vi "TagSyncFPGA.vi"() -> ()   [LabVIEW 2017]
uses:
  <vilib>/rvi/Emulation/niFpgaSctlEmulationGetInTimedLoop.vi
  <vilib>/rvi/Emulation/niFpgaProcessEmulError.vi
  <vilib>/rvi/Emulation/niFpgaGetClockAttributes.vi
  <vilib>/rvi/Emulation/niFpgaEmulationReportErrorSimple.vi
  <vilib>/rvi/Emulation/niFpgaCriticalErrorInLSC.vi
  <vilib>/rvi/eio/common/nirviEmuTemplateMethod_errors.vi
  <vilib>/eio/EIONode/EIONode.xnode
panel:
  in  "Sync Tagging":T1(tab)
  out "Minimum tagging period (pws)":u32=87
  out "Total tag data length (pws)":u32=86
  in  "TaggingPeriod (pws)":u32=100
  out "TagMarkerDuration (pws)":u16=10
  in  "PulseWidth (ms)":u32=10
  out "Tag data does NOT fit in period!!!":bool
  in  "Halt tagging":bool
  out "Tag monitor":i16(graph)
  in  "Enable monitoring":bool
  out "Current tag number":i32=665
  out "Tag data":bool[](array[boolean])=[TRUE, TRUE, TRUE, TRUE, TRUE, TRUE, TRUE, TRUE, TRUE, TRUE, FALSE, TRUE, FALSE, FALSE, FALSE, FALSE, FALSE, TRUE, FALSE, TRUE, FALSE, FALSE, FALSE, FALSE, FALSE, TRUE, FALSE, FALSE, FALSE, TRUE, FALSE, FALSE, FALSE, FALSE, FALSE, FALSE, FALSE, FALSE, FALSE, FALSE, FALSE, FALSE, FALSE, FALSE, FALSE, FALSE, FALSE, FALSE, FALSE, FALSE, FALSE, FALSE, FALSE, FALSE, FALSE, FALSE, FALSE, FALSE, FALSE, FALSE, FALSE, FALSE, FALSE, FALSE, FALSE, FALSE, FALSE, FALSE, FALSE, FALSE, FALSE, FALSE, FALSE, FALSE, FALSE, FALSE, TRUE, TRUE, TRUE, TRUE, TRUE, TRUE, TRUE, TRUE, TRUE, TRUE, FALSE, FALSE, FALSE, FALSE, FALSE, FALSE, FALSE, FALSE, FALSE, FALSE, FALSE, FALSE, FALSE, FALSE, FALSE, FALSE, FALSE, FALSE, FALSE, FALSE, FALSE, FALSE, FALSE, FALSE, FALSE, FALSE, FALSE, FALSE, FALSE, FALSE, FALSE, FALSE, FALSE, FALSE, FALSE, FALSE, FALSE, FALSE, FALSE, FALSE, FALSE, FALSE, FALSE, FALSE, FALSE, FALSE, FALSE, FALSE, FALSE, FALSE, FALSE, FALSE, FALSE, FALSE, FALSE, FALSE, FALSE, FALSE, FALSE, FALSE, FALSE, FALSE, FALSE, FALSE, FALSE, FALSE]
  out "SyncTagOutput":bool
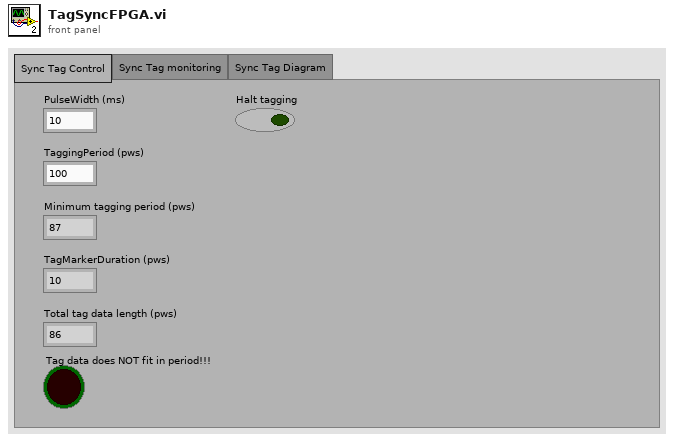
[diagram p1: front panel]
types:
  T1 = enum32{"Sync Tag Control", "Sync Tag monitoring", "Sync Tag Diagram"}
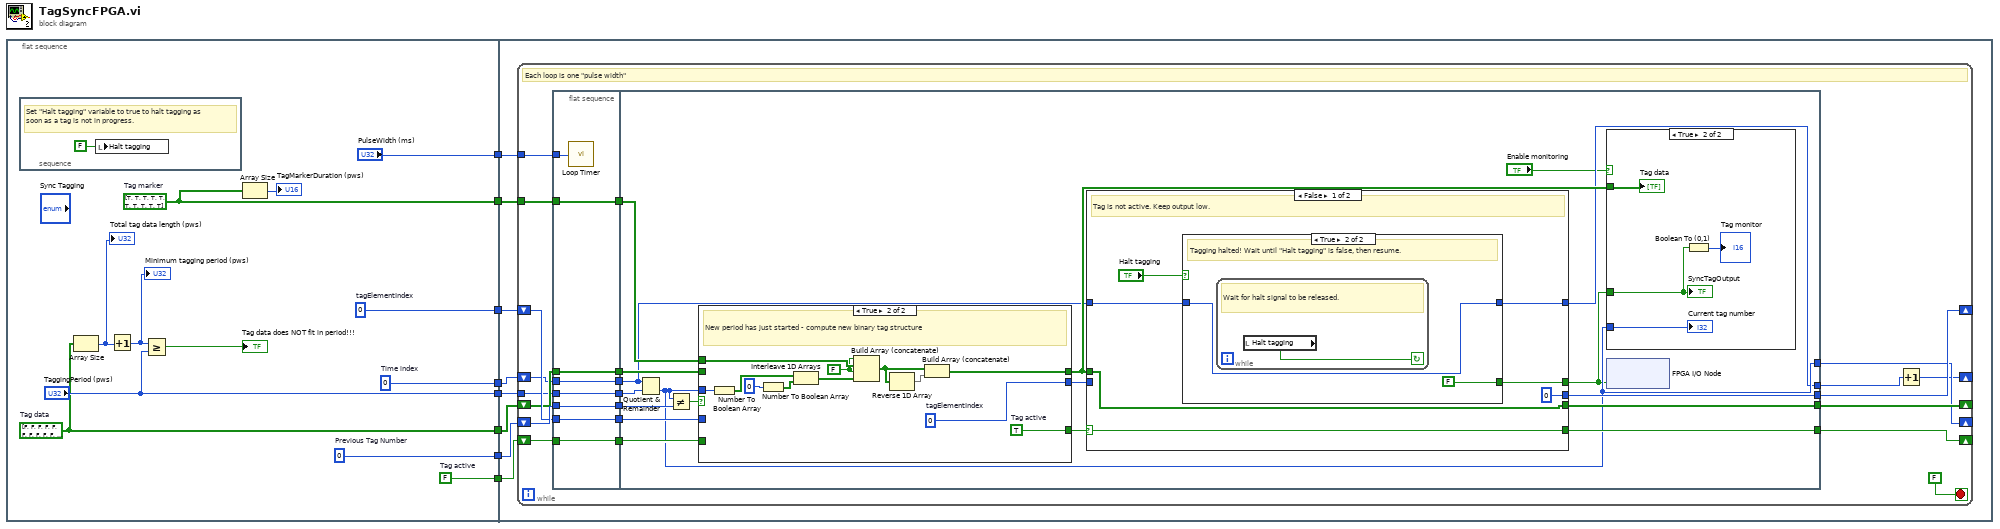
[diagram p0: block diagram]
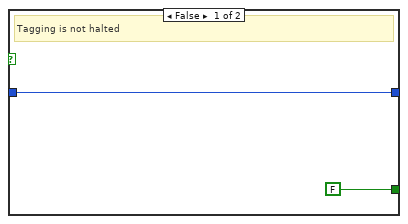
[diagram p3: hidden frame]
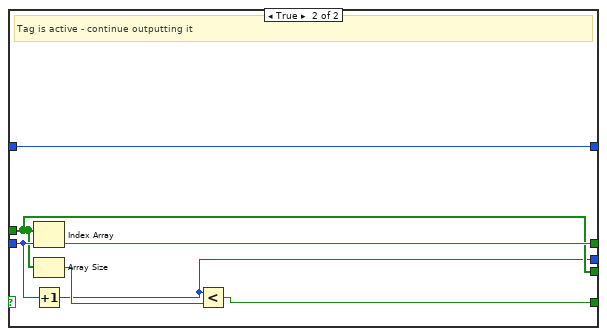
[diagram p4: hidden frame]
diagram:
  n1 = flat-sequence {
    tunnel: ["TaggingPeriod (pws)"] -> w8
    tunnel: [w19] -> w7
    tunnel: [w18] -> w6
    tunnel: [w17] -> w5
    tunnel: [w16] -> w4
    tunnel: [w15] -> w3
    tunnel: ["PulseWidth (ms)"] -> w2
    tunnel: [w13] -> w1
    tunnel: w8 -> [w25]
    tunnel: w7 -> [w24]
    tunnel: w6 -> [w28]
    tunnel: w5 -> [w26]
    tunnel: w4 -> [w27]
    tunnel: w3 -> [w29]
    tunnel: w2 -> [w23]
    tunnel: w1 -> [w22]
    frame #0 {
      w13 = u32 0  # Time index
      w19 = bool[] [TRUE, TRUE, TRUE, TRUE, TRUE, TRUE, TRUE, TRUE, TRUE, TRUE]  # Tag marker
      w17 = u32 0  # tagElementIndex
      w16 = FALSE  # Tag active
      w18 = bool[] [FALSE, FALSE, FALSE, FALSE, FALSE, FALSE, FALSE, FALSE, FALSE, FALSE, FALSE, FALSE, FALSE, FALSE, FALSE, FALSE, FALSE, FALSE, FALSE, FALSE, FALSE, FALSE, FALSE, FALSE, FALSE, FALSE, FALSE, FALSE, FALSE, FALSE, FALSE, FALSE, FALSE, FALSE, FALSE, FALSE, FALSE, FALSE, FALSE, FALSE, FALSE, FALSE, FALSE, FALSE, FALSE, FALSE, FALSE, FALSE, FALSE, FALSE, FALSE, FALSE, FALSE, FALSE, FALSE, FALSE, FALSE, FALSE, FALSE, FALSE, FALSE, FALSE, FALSE, FALSE, FALSE, FALSE, FALSE, FALSE, FALSE, FALSE, FALSE, FALSE, FALSE, FALSE, FALSE, FALSE, FALSE, FALSE, FALSE, FALSE, FALSE, FALSE, FALSE, FALSE, FALSE, FALSE, FALSE, FALSE, FALSE, FALSE, FALSE, FALSE, FALSE, FALSE, FALSE, FALSE, FALSE, FALSE, FALSE, FALSE, FALSE, FALSE, FALSE, FALSE, FALSE, FALSE, FALSE, FALSE, FALSE, FALSE, FALSE, FALSE, FALSE, FALSE, FALSE, FALSE, FALSE, FALSE, FALSE, FALSE, FALSE, FALSE, FALSE, FALSE, FALSE, FALSE, FALSE, FALSE, FALSE, FALSE, FALSE, FALSE, FALSE, FALSE, FALSE, FALSE, FALSE, FALSE, FALSE, FALSE, FALSE, FALSE, FALSE, FALSE, FALSE, FALSE, FALSE, FALSE, FALSE, FALSE, FALSE, FALSE]  # Tag data
      w15 = u32 0  # Previous Tag Number
      n2 = stacked-sequence {
        frame #0 {
          # "Set \"Halt tagging\" variable to true to halt tagging as soon as a tag is not in progress."
          n3 = local write "Halt tagging"(FALSE ("Halt tagging")) -> ()
        }
      }
      n4 = Array Size(array=w18) -> (size(s)=w12:i32)
      "Total tag data length (pws)" <- w12
      n5 = Increment(x=w12) -> (x+1=w9:i32)
      "Minimum tagging period (pws)" <- w9
      n6 = Greater Or Equal?(x=w9, y="TaggingPeriod (pws)") -> (x >= y?=→"Tag data does NOT fit in period!!!":bool)
      n7 = Array Size(array=w19) -> (size(s)=→"TagMarkerDuration (pws)":i32)
    }
    frame #1 {
      n8 = while {
        shift-right: [w42] -> _
        shift-left: w29 -> [w51]
        shift-right: [w48] -> _
        shift-left: w28 -> [w45]
        shift-right: [w46] -> _
        shift-left: w27 -> [w50]
        shift-right: [w47] -> _
        shift-left: w26 -> [w49]
        tunnel: w25 -> [w44]
        tunnel: w24 -> [w43]
        tunnel: w23 -> [w35]
        shift-right: [w31] -> _
        shift-left: w22 -> [w33]
        stop <- FALSE stop-if-true
        # "Each loop is one \"pulse width\""
        n9 = flat-sequence {
          tunnel: w43 -> [w54]
          tunnel: w44 -> [w55]
          tunnel: w45 -> [w56]
          tunnel: w49 -> [w57]
          tunnel: w50 -> [w58]
          tunnel: w51 -> [w59]
          tunnel: [w59] -> w41
          tunnel: [w58] -> w40
          tunnel: [w57] -> w39
          tunnel: [w56] -> w38
          tunnel: [w55] -> w37
          tunnel: [w54] -> w36
          tunnel: w35 -> [w52]
          tunnel: w33 -> [w53]
          tunnel: [w53] -> w32
          tunnel: w41 -> [w77]
          tunnel: w40 -> [w75]
          tunnel: w39 -> [w73]
          tunnel: w38 -> [w68]
          tunnel: w37 -> [w67]
          tunnel: w36 -> [w66]
          tunnel: w32 -> [w64]
          tunnel: [w71] -> w48
          tunnel: [w70] -> w47
          tunnel: [w69] -> w46
          tunnel: [w63] -> w42
          tunnel: [w62] -> w30
          frame #0 {
            n10 = call "Loop Timer"("Count(mSec)"=w52) -> ()  [unwired: 1 out]
          }
          frame #1 {
            n11 = Quotient & Remainder(x=w64, y=w67) -> (floor(x/y)=w63:u32)  [unwired: 1 out]
            n12 = Not Equal?(x=w63, y=w77) -> (x != y?=w76:bool)
            n13 = case shown="True" w76 {
              tunnel: w63 -> [_ w115]
              tunnel: w68 -> [w103 _]
              tunnel: w75 -> [w101 _]
              tunnel: [w101 w114] -> w74
              tunnel: [w103 w104] -> w65
              tunnel: w73 -> [w102 _]
              tunnel: [w102 w109] -> w72
              tunnel: w66 -> [_ w108]
              frame False {
              }
              frame True {
                w109 = u16 0  # tagElementIndex
                w107 = FALSE ("Marker on")
                w114 = TRUE  # Tag active
                # "New period has just started - compute new binary tag structure"
                n14 = Number To Boolean Array(number=w115) -> (Boolean array=w112:bool[])
                n15 = Number To Boolean Array(number=0) -> (Boolean array=w111:bool[])
                n16 = Interleave 1D Arrays(w112, w111) -> (w110:bool[])
                n17 = Build Array (concatenate)(w107, w108, w107, w110) -> (w105:bool[])
                n18 = Reverse 1D Array(array=w105) -> (reversed array=w106:bool[])
                n19 = Build Array (concatenate)(w105, w106) -> (w104:bool[])
              }
            }
            n20 = case shown="False" w74 {
              selector: w74 -> [w86 _]
              tunnel: w65 -> [w88 w97]
              tunnel: [w88 w97] -> w71
              tunnel: w72 -> [_ w100]
              tunnel: [u16 0 w96] -> w70
              tunnel: [w87 w99] -> w61
              tunnel: [w86 w95] -> w69
              tunnel: [w84 w94] -> w62
              tunnel: w64 -> [w83 w94]
              frame False {
                # "Tag is not active. Keep output low."
                n21 = case shown="True" "Halt tagging" {
                  tunnel: [FALSE ("Output 2") FALSE ("Output 2")] -> w87
                  tunnel: w83 -> [w90 w91]
                  tunnel: [w90 w91] -> w84
                  frame False {
                    # "Tagging is not halted"
                  }
                  frame True {
                    # "Tagging halted! Wait until \"Halt tagging\" is false, then resume."
                    n22 = while {
                      stop <- w93 continue-if-true
                      # "Wait for halt signal to be released."
                      n23 = local read "Halt tagging"() -> (w93:bool)
                    }
                  }
                }
              }
              frame True {
                # "Tag is active - continue outputting it"
                n24 = Index Array(array=w97, index=w100) -> (element=w99:bool)
                n25 = Array Size(array=w97) -> (size(s)=w98:i32)
                n26 = Increment(x=w100) -> (x+1=w96:u32)
                n27 = Less?(x=w96, y=w98) -> (x < y?=w95:bool)
              }
            }
            n28 = case shown="True" "Enable monitoring" {
              tunnel: w65 -> [_ w81]
              tunnel: w61 -> [_ w78]
              tunnel: w63 -> [_ w79]
              frame False {
              }
              frame True {
                n29 = Boolean To (0,1)(Boolean=w78) -> (0, 1=→"Tag monitor":i16)
                "Current tag number" <- w79
                "Tag data" <- w81
                "SyncTagOutput" <- w78
              }
            }
            n30 = xnode "FPGA I/O Node"("DIO7"=w61) -> ()  [unwired: 1 in, 1 out]
          }
        }
        n31 = Increment(x=w30) -> (x+1=w31:u32)
      }
    }
  }
